vi "Configure VIs for Execution.vi"   [LabVIEW 2016, in "Static Error Handling.lvlib"]
uses:
  Static Error Handling.lvlib
types:
  T1 = enum32{"invalid VI type", "Standard VI", "Control VI", "Global VI", "Polymorphic VI", "Configuration VI", "SubSystem", "Facade VI", "Method VI", "Statechart Diagram VI"}
  T2 = enum16{"Share clones between instances", "Preallocate clone for each instance"}
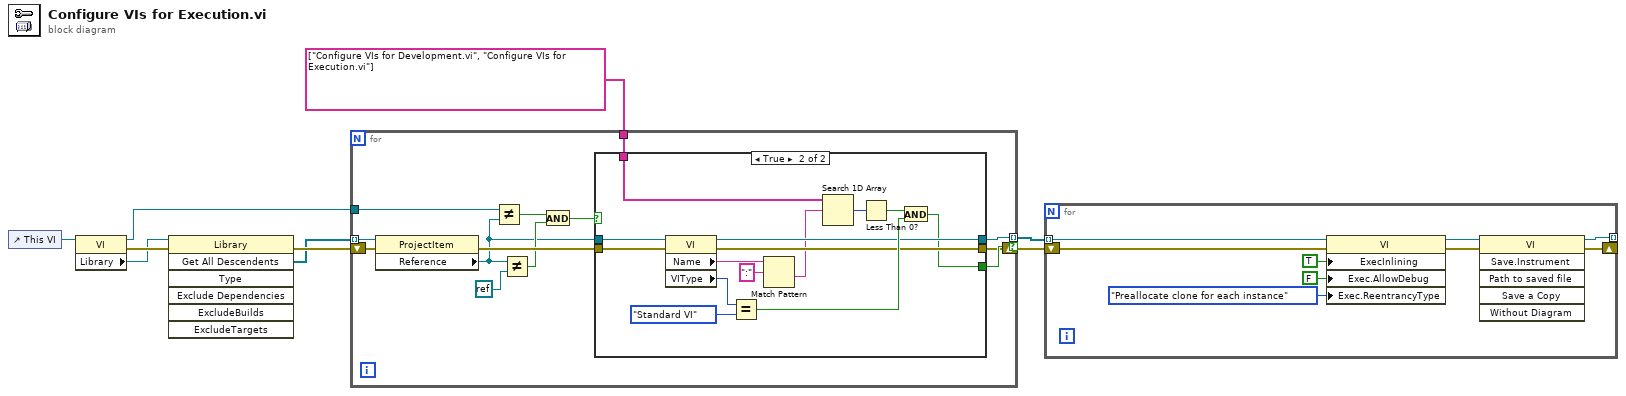
[diagram p0: block diagram]
diagram:
  n1 = control-ref of="This VI"() -> (w9:refnum<vi>)
  n2 = property class="VI"(reference=w9) -> (reference out=w8:refnum<vi>, error out=w2:errorcluster, "Library"=w1:refnum<vi>)  [unwired: 1 in]
  n3 = invoke class="Library" method="Get All Descendents"(reference=w1, error in=w2) -> (error out=w6:errorcluster, "All Descendents"=w5:refnum<vi>[])  [unwired: 5 in, 5 out]
  n4 = for {
    tunnel: w5 -> [w22] mode=indexing
    tunnel: [w21] -> w4 mode=indexing if=w20
    tunnel: w8 -> [w18]
    shift-right: [w16] -> w7
    shift-left: w6 -> [w15]
    tunnel: string[] ["Configure VIs for Development.vi", "Configure VIs for Execution.vi"] ("Blacklist VIs") -> [w10]
    n5 = property class="ProjectItem"(reference=w22, error in=w15) -> (error out=w14:errorcluster, "Reference"=w11:refnum<vi>)  [unwired: 1 out]
    n6 = Not Equal?(x=w18, y=w11) -> (x != y?=w17:bool)
    n7 = Not Equal?(x=w11, y=refnum<k0> refnum) -> (x != y?=w13:bool)
    n8 = And(x=w17, y=w13) -> (x .and. y?=w12:bool)
    n9 = case shown="True" w12 {
      selector: w12 -> [w24 _]
      tunnel: [w25 w30] -> w21
      tunnel: [w24 w27] -> w20
      tunnel: w11 -> [w25 w31]
      tunnel: [w23 w29] -> w16
      tunnel: w14 -> [w23 w32]
      tunnel: w10 -> [_ w28]
      frame False {
      }
      frame True {
        n10 = property class="VI"(reference=w31, error in=w32) -> (reference out=w30:refnum<vi>, error out=w29:errorcluster, "Name"=w33:string, "VIType"=w38:T1)
        n11 = Equal?(x=w38, y=T1."Standard VI" ("VI Type")) -> (x = y?=w35:bool)
        n12 = Match Pattern(string=w33, regular expression=":") -> (after substring=w26:string)  [unwired: 1 in, 3 out]
        n13 = Search 1D Array(1D array=w28, element=w26) -> (index of element=w37:i32)  [unwired: 1 in]
        n14 = Less Than 0?(x=w37) -> (x < 0?=w36:bool)
        n15 = And(x=w36, y=w35) -> (x .and. y?=w27:bool)
      }
    }
  }
  n16 = for {
    tunnel: w4 -> [w48] mode=indexing
    tunnel: [w40] -> _ mode=indexing
    shift-right: [w41] -> _
    shift-left: w7 -> [w47]
    n17 = property class="VI"(reference=w48, error in=w47, "ExecInlining"=TRUE ("Execution:Inline SubVI"), "Exec.AllowDebug"=FALSE ("Execution:Allow Debugging"), "Exec.ReentrancyType"=T2."Preallocate clone for each instance" ("Execution:Reentrancy Type")) -> (reference out=w42:refnum<vi>, error out=w43:errorcluster)
    n18 = invoke class="VI" method="Save.Instrument"(reference=w42, error in=w43) -> (reference out=w40:refnum<vi>, error out=w41:errorcluster)  [unwired: 4 in, 4 out]
  }
